vi "Write Measurement RefreshTime (ms).vi"(8 "error in (no error)":errorcluster, 10 "Measurement RefreshTime (ms)":u32, 11 "SiemensDigitalEnergyMeter in":refnum<class "SiemensDigitalEnergyMeter.lvclass">) -> (0 "error out":errorcluster, 3 "SiemensDigitalEnergyMeter out":refnum<class "SiemensDigitalEnergyMeter.lvclass">)   [LabVIEW 2018, in "SensorPlugins.lvlib" / "SiemensDigitalEnergyMeter.lvclass"]
uses:
  SiemensDigitalEnergyMeter.lvclass
  SiemensDigitalEnergyMeter.lvclass/SiemensDigitalEnergyMeter.ctl
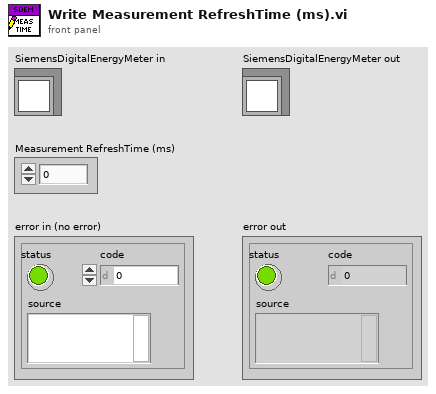
[diagram p1: front panel]
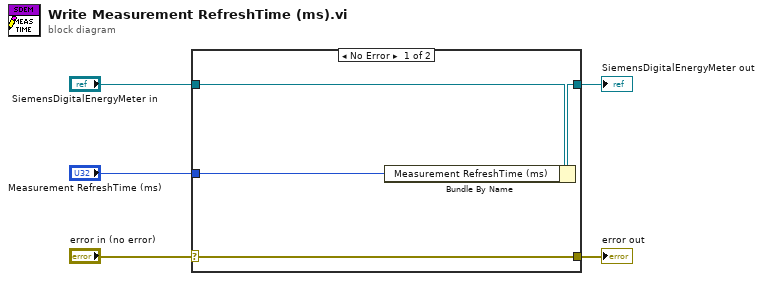
[diagram p0: block diagram]
diagram:
  n1 = case shown="No Error" "error in (no error)" {
    selector: "error in (no error)" -> [w9 w10]
    tunnel: [w9 w10] -> w4
    tunnel: [w7 w11] -> w2
    tunnel: "SiemensDigitalEnergyMeter in" -> [w8 w11]
    tunnel: "Measurement RefreshTime (ms)" -> [w6 _]
    frame No Error {
      n2 = Bundle By Name(cluster=w8, "Measurement RefreshTime (ms)"=w6) -> (w7:refnum<class "SiemensDigitalEnergyMeter.lvclass">)
    }
    frame Error {
    }
  }
  "error out" <- w4
  "SiemensDigitalEnergyMeter out" <- w2
